vi "Utility Reset.vi"(5 "Retry Attempts (0)":i32 min=0, 8 "error in (no error)":errorcluster, 10 "Fast Comms (F)":bool, 11 "VISA resource name":refnum<visa-resource-name>) -> (0 "error out":errorcluster, 3 "VISA resource name out":refnum<visa-resource-name>)   [LabVIEW 2020, in "driver_chromtech_next_gen.lvlib"]
doc: "Resets the instrument and then sends a set of default setup commands to the instrument."
uses:
  driver_chromtech_next_gen.lvlib
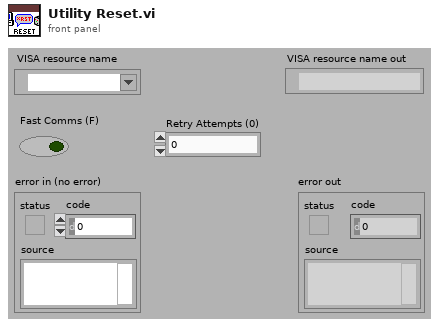
[diagram p1: front panel]
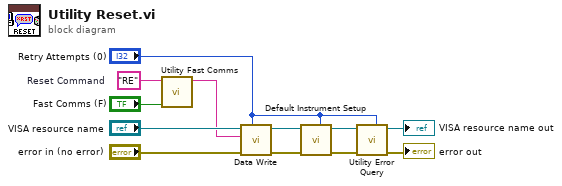
[diagram p0: block diagram]
diagram:
  w3 = "RE"  # Reset Command
  n1 = call "Utility Fast Comms.vi"("Fast Comms"="Fast Comms (F)", "Command"=w3) -> ("Fast Command"=w2:string)  [unwired: 9 in]
  n2 = call "Data Write.vi"("Retry Attempts (0)"="Retry Attempts (0)", "error in (no error)"="error in (no error)", "Command"=w2, "VISA Refnum in"="VISA resource name") -> ("error out"=w10:errorcluster, "VISA Refnum out"=w9:refnum<visa-resource-name>)  [unwired: 6 in]
  n3 = call "Default Instrument Setup.vi"("Retry Attempts (0)"="Retry Attempts (0)", "error in (no error)"=w10, "VISA resource name"=w9) -> ("error out"=w8:errorcluster, "VISA resource name out"=w7:refnum<visa-resource-name>)  [unwired: 7 in]
  n4 = call "Utility Error Query.vi"("Retry Attempts (0)"="Retry Attempts (0)", "error in (no error)"=w8, "VISA resource name"=w7) -> ("error out"=→"error out":errorcluster, "VISA resource name out"=→"VISA resource name out":refnum<visa-resource-name>)  [unwired: 5 in, 2 out]
